vi "Init.vi"(4 "Base Path":path, 6 "Template Name":string, 8 "Project:Active Project":refnum<vi>, 9 "Application Instance":refnum<vi>, 10 "Name":string, 11 "Actor Script Strategy in":refnum<class "Actor Script Strategy.lvclass">) -> (3 "Actor Script Strategy out":refnum<class "Actor Script Strategy.lvclass">)   [LabVIEW 2021, in "_Template.lvlib" / "Script Strategy.lvlib" / "Actor Script Strategy.lvclass"]
uses:
  Actor Script Strategy.lvclass
  Actor Script Strategy.lvclass/Actor Script Strategy.ctl
  _Template.lvlib
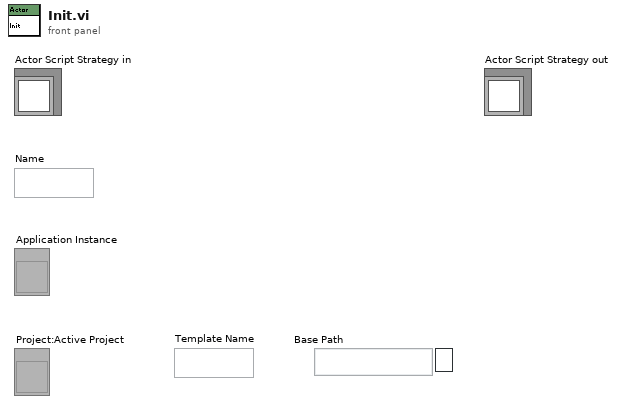
[diagram p1: front panel]
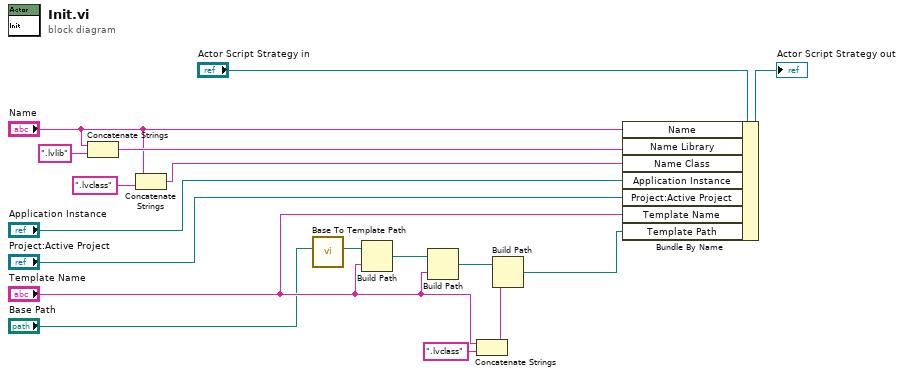
[diagram p0: block diagram]
diagram:
  n1 = Concatenate Strings("Name", ".lvlib" ("string")) -> (w15:string)
  n2 = Concatenate Strings("Name", ".lvclass" ("regular expression")) -> (w13:string)
  n3 = call "Base To Template Path.vi"("Base Path"="Base Path") -> ("Templates Path"=w6:path)  [unwired: 10 in]
  n4 = Build Path(base path=w6, name or relative path="Template Name") -> (appended path=w5:path)
  n5 = Build Path(base path=w5, name or relative path="Template Name") -> (appended path=w4:path)
  n6 = Concatenate Strings("Template Name", ".lvclass" ("string")) -> (w7:string)
  n7 = Build Path(base path=w4, name or relative path=w7) -> (appended path=w1:path)
  n8 = Bundle By Name(cluster="Actor Script Strategy in", "Name"="Name", "Name Library"=w15, "Name Class"=w13, "Application Instance"="Application Instance", "Project:Active Project"="Project:Active Project", "Template Name"="Template Name", "Template Path"=w1) -> (→"Actor Script Strategy out":refnum<class "Actor Script Strategy.lvclass">)
